vi "Periodic Tasks.vi"(8 "error in":errorcluster) -> ()   [LabVIEW 2023]
doc: "This VI runs in parallel to other tasks. It can contain as many user-defined periodic loops as you need. These can carry out PID or other sorts of timed response."
uses:
  <vilib>/Rock Robotics/WPI/ThirdParty/Phoenix-LabVIEW/Motor Controller/Controls/CTRE_Phoenix_MotorControl_ControlMode.ctl
  <vilib>/Rock Robotics/WPI/Utilities/WPI_GetSetVariantRefNum.vi
  <vilib>/Rock Robotics/Network Tables/NT Read Number.vi
  <vilib>/Rock Robotics/Network Tables/NT Write Boolean.vi
  Robot Global Data.vi
panel:
  out "In Range Speaker Right?":bool=TRUE
  out "In Range Speaker Left?":bool=TRUE
  out "In Range Center?":bool=TRUE
  out "Values":T1
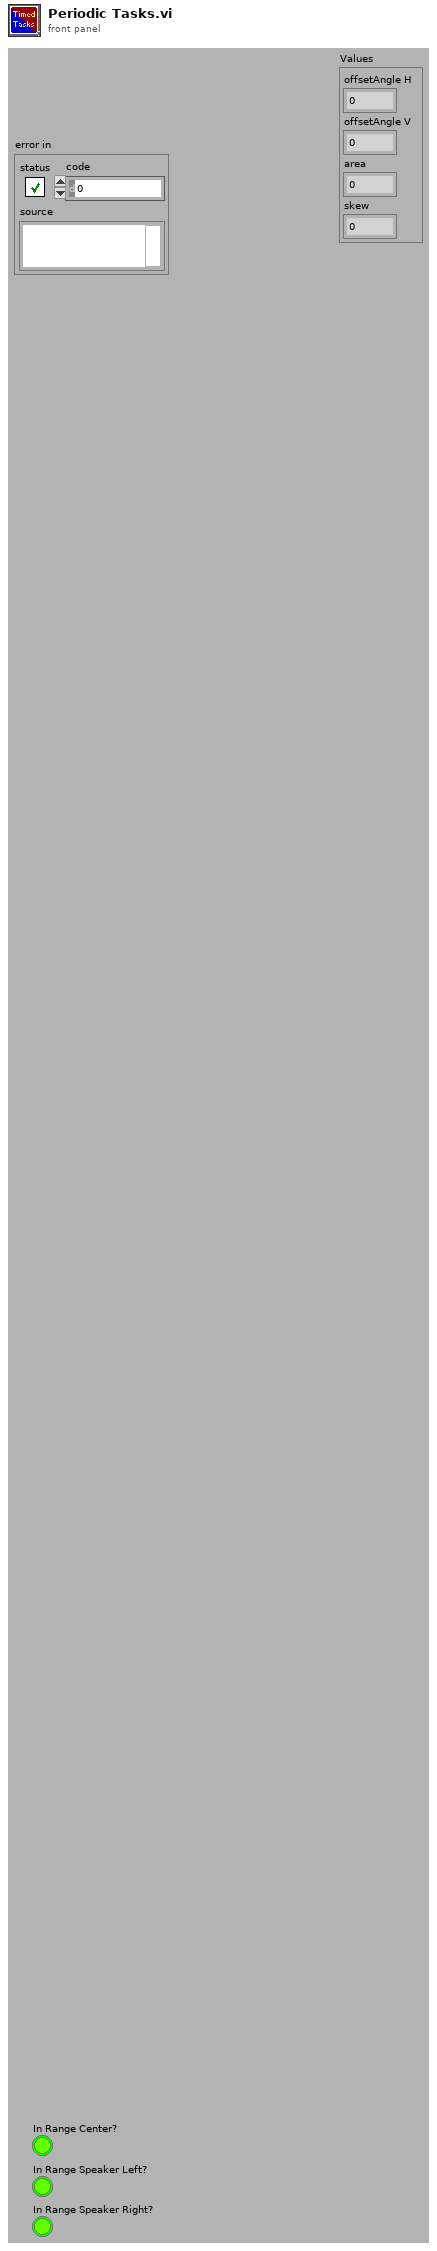
[diagram p1: front panel]
types:
  T1 = cluster{"offsetAngle H":dbl, "offsetAngle V":dbl, "area":dbl, "skew":dbl}
  T2 = typedef "WPI_JoystickDevRef.ctl" = cluster{"Device":T3}
  T3 = typedef "WPI_JoystickDeviceEnum.ctl" = enum16{"USB 0", "USB 1", "USB 2", "USB 3", "USB 4", "USB 5"}
  T4 = typedef "WPI_RobotDriveDevRef.ctl" = cluster{"DevStatus":errorcluster, "Motors[]":T5[], "Square Inputs":bool, "Max Output":dbl}
  T5 = typedef "WPI_MotorControlDeviceRef.ctl" = cluster{"DeviceStatus":errorcluster, "Type":T6, "PWM":cluster{"PWM Channel":T7, "DeadBand":T8}, "CAN":cluster{"Device Number":u8, "SetOutput VI Ref":variant, "GetOutput VI Ref":variant, "Enable VI Ref":variant, "Disable VI Ref":variant, "Data":variant}, "Invert":bool, "DIO PWM":cluster{"PWM \"Enable\" Channel":T7, "DIOChannel":T9, "PWM Rate":dbl}}
  T6 = typedef "WPI_MotorControlType.ctl" = enum16{"PWM", "CAN", "DIO PWM"}
  T7 = typedef "FPGA_DIOPWMChannel.ctl" = enum8{"PWM 0", "PWM 1", "PWM 2", "PWM 3", "PWM 4", "PWM 5", "PWM 6", "PWM 7", "PWM 8", "PWM 9", "PWM MXP 0", "PWM MXP 1", "PWM MXP 2", "PWM MXP 3", "PWM MXP 4", "PWM MXP 5", "PWM MXP 6", "PWM MXP 7", "PWM MXP 8", "PWM MXP 9", "Invalid"}
  T8 = typedef "WPI_PWMDeadband.ctl" = cluster{"Name":string, "maxPositivePwm":i32, "minPositivePwm":i32, "centerPwm":i32, "maxNegativePwm":i32, "minNegativePwm":i32, "angularRange":u16}
  T9 = typedef "FPGA_DIOChannel.ctl" = enum8{"DIO 0", "DIO 1", "DIO 2", "DIO 3", "DIO 4", "DIO 5", "DIO 6", "DIO 7", "DIO 8", "DIO 9", "DIO MXP 0", "DIO MXP 1", "DIO MXP 2", "DIO MXP 3", "DIO MXP 4", "DIO MXP 5", "DIO MXP 6", "DIO MXP 7", "DIO MXP 8", "DIO MXP 9", "DIO MXP 10", "DIO MXP 11", "DIO MXP 12", "DIO MXP 13", "DIO MXP 14", "DIO MXP 15", "SPI Port CS1", "SPI Port CS2", "SPI Port CS3", "SPI Port MISO", "SPI Port MOSI", "Invalid"}
  T10 = cluster{"JoystickDevRef":T2, "RobotDriveDevRef":T4}
  T11 = typedef "CTRE_Phoenix_MotorControl_ControlMode.ctl" = u16
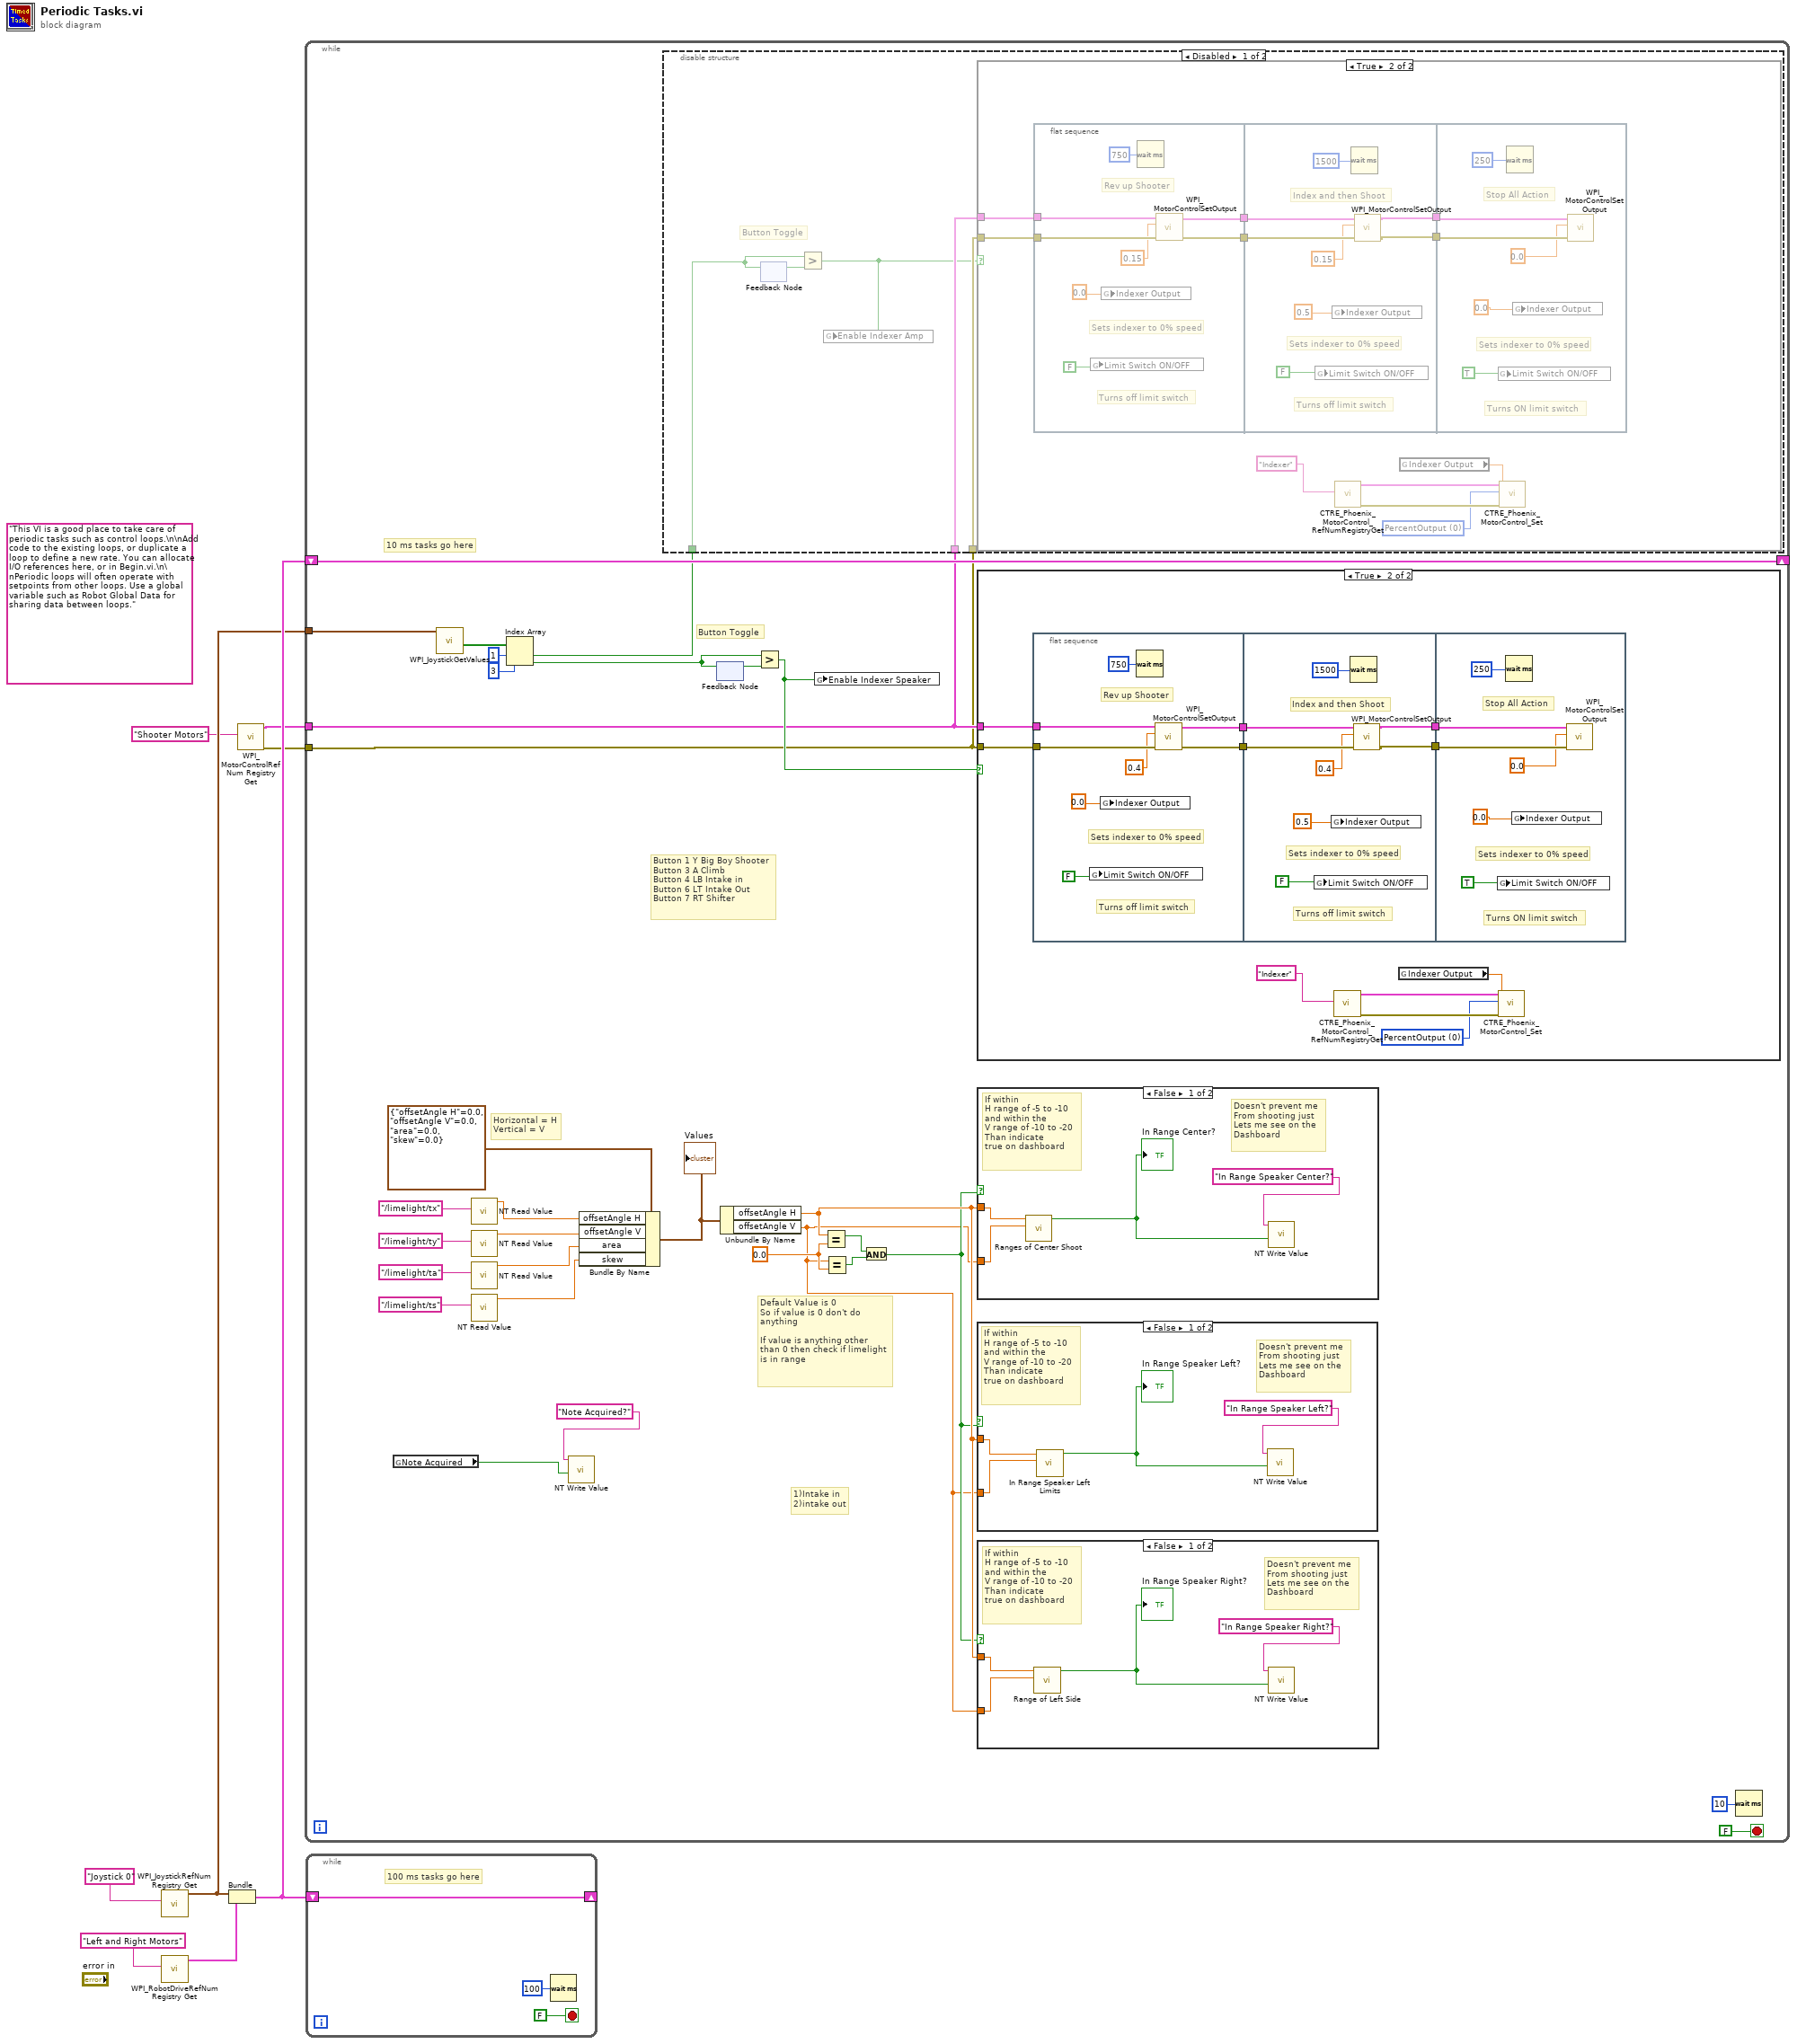
[diagram p0: block diagram]
diagram:
  (unwired) "This VI is a good place to take care of periodic tasks such as control loops.\n\nAdd code to the existing loops, or duplicate a loop to define a new rate. You can allocate I/O references here, or in Begin.vi.\n\nPeriodic loops will often operate with setpoints from other loops. Use a global variable such as Robot Global Data for sharing data between loops."
  n1 = call <vilib>:"WPI_JoystickRefNum Registry Get.vi"("refnum name"="Joystick 0") -> ("JoystickDevRef"=w4:T2)  [unwired: 1 in, 9 out]
  n2 = call <vilib>:"WPI_RobotDriveRefNum Registry Get.vi"("refnum name"="Left and Right Motors") -> ("RobotDriveDevRef"=w6:T4)  [unwired: 1 in, 9 out]
  n3 = Bundle("JoystickDevRef"=w4, "RobotDriveDevRef"=w6) -> (w5:T10)  [unwired: 1 out]
  n4 = call <vilib>:"WPI_MotorControlRefNum Registry Get.vi"("refnum name"="Shooter Motors") -> ("error out"=w1:errorcluster, "MotorControlDevRef"=w2:T5)  [unwired: 9 in]
  n5 = while {
    shift-right: [w37] -> _
    shift-left: w5 -> [w37]
    tunnel: w4 -> [w33]
    tunnel: w2 -> [w15]
    tunnel: w1 -> [w14]
    stop <- FALSE stop-if-true
    w19 = 0.0 ("y")
    # "1)Intake in\n2)intake out"
    # "Default Value is 0\nSo if value is 0 don't do\nanything\n\nIf value is anything other \nthan 0 then check if limelight\nis in range"
    # "Horizontal = H\nVertical = V"
    # "Button 1 Y Big Boy Shooter\nButton 3 A Climb\nButton 4 LB Intake in\nButton 6 LT Intake Out\nButton 7 RT Shifter"
    # "Button Toggle"
    # "10 ms tasks go here"
    n6 = global read "Robot Global Data.vi" "Note Acquired"() -> (w9:bool)
    n7 = call <vilib>:"WPI_JoystickGetValues.vi"("JoystickDevRef"=w33) -> ("Buttons"=w36:bool[])  [unwired: 6 in, 4 out]
    n8 = call-poly <vilib>:"NT Read Value.vi"("name"="/limelight/tx") -> ("value"=w25:dbl)  [unwired: 8 in, 2 out]
    n9 = call-poly <vilib>:"NT Read Value.vi"("name"="/limelight/ty") -> ("value"=w24:dbl)  [unwired: 8 in, 2 out]
    n10 = call-poly <vilib>:"NT Read Value.vi"("name"="/limelight/ta") -> ("value"=w27:dbl)  [unwired: 8 in, 2 out]
    n11 = call-poly <vilib>:"NT Read Value.vi"("name"="/limelight/ts") -> ("value"=w26:dbl)  [unwired: 8 in, 2 out]
    n12 = Index Array(array=w36, index #1=1 ("index"), index #2=3 ("index")) -> (element #1=w12:bool, element #2=w13:bool)
    n13 = call-poly <vilib>:"NT Write Value.vi"("value"=w9, "name"="Note Acquired?") -> ()  [unwired: 9 in, 1 out]
    n14 = Bundle By Name(cluster=T1 {"offsetAngle H"=0.0, "offsetAngle V"=0.0, "area"=0.0, "skew"=0.0}, "offsetAngle H"=w25, "offsetAngle V"=w24, "area"=w27, "skew"=w26) -> (w23:T1)
    "Values" <- w23
    n15 = disable-structure shown="Disabled" {
      disable-tunnel: w15 -> [w44 _]
      disable-tunnel: w14 -> [w43 _]
      disable-tunnel: w12 -> [w41 _]
      frame Disabled {
        # "Button Toggle"
        n16 = feedback #1() -> (w42:bool)  [unwired: 1 in]
        n17 = feedback-in #1(w41) -> ()
        n18 = Greater?(x=w41, y=w42) -> (0:w40:bool)
        n19 = global write "Robot Global Data.vi" "Enable Indexer Amp"(w40) -> ()
        n20 = case shown="True" w40 {
          tunnel: w44 -> [_ w55]
          tunnel: w43 -> [_ w54]
          frame False {
          }
          frame True {
            w46 = T11 0 items=["PercentOutput"=0, "Position"=1, "Velocity"=2, "Current"=3, "Follower"=5, "MotionProfile"=6, "MotionMagic"=7, "MotionProfileArc"=10, "Disabled"=15] ("Control Mode")
            n21 = flat-sequence {
              tunnel: [w60] -> w53
              tunnel: [w59] -> w52
              tunnel: w55 -> [w63]
              tunnel: w54 -> [w62]
              tunnel: w53 -> [w70]
              tunnel: w52 -> [w69]
              tunnel: [w68] -> w51
              tunnel: [w67] -> w50
              tunnel: w51 -> [w77]
              tunnel: w50 -> [w76]
              frame #0 {
                # "Sets indexer to 0% speed"
                # "Rev up Shooter"
                # "Turns off limit switch"
                n22 = global write "Robot Global Data.vi" "Limit Switch ON/OFF"(FALSE ("Limit Switch ON/OFF")) -> ()
                n23 = global write "Robot Global Data.vi" "Indexer Output"(0.0 ("Indexer Output")) -> ()
                n24 = Wait (ms)(milliseconds to wait=u32 750) -> ()  [unwired: 1 out]
                n25 = call <vilib>:"WPI_MotorControlSetOutput.vi"("error in (no error)"=w62, "Output"=0.15, "MotorControlDevRef"=w63) -> ("error out"=w59:errorcluster, "MotorControlDevRef"=w60:T5)  [unwired: 6 in, 1 out]
              }
              frame #1 {
                # "Sets indexer to 0% speed"
                # "Turns off limit switch"
                # "Index and then Shoot"
                n26 = global write "Robot Global Data.vi" "Limit Switch ON/OFF"(FALSE ("Limit Switch ON/OFF")) -> ()
                n27 = global write "Robot Global Data.vi" "Indexer Output"(0.5 ("Indexer Output")) -> ()
                n28 = Wait (ms)(milliseconds to wait=u32 1500) -> ()  [unwired: 1 out]
                n29 = call <vilib>:"WPI_MotorControlSetOutput.vi"("error in (no error)"=w69, "Output"=0.15, "MotorControlDevRef"=w70) -> ("error out"=w67:errorcluster, "MotorControlDevRef"=w68:T5)  [unwired: 6 in, 1 out]
              }
              frame #2 {
                # "Sets indexer to 0% speed"
                # "Turns ON limit switch"
                # "Stop All Action"
                n30 = global write "Robot Global Data.vi" "Limit Switch ON/OFF"(TRUE ("Limit Switch ON/OFF")) -> ()
                n31 = Wait (ms)(milliseconds to wait=u32 250) -> ()  [unwired: 1 out]
                n32 = global write "Robot Global Data.vi" "Indexer Output"(0.0 ("Indexer Output")) -> ()
                n33 = call <vilib>:"WPI_MotorControlSetOutput.vi"("error in (no error)"=w76, "Output"=0.0, "MotorControlDevRef"=w77) -> ()  [unwired: 6 in, 3 out]
              }
            }
            n34 = call <vilib>:"CTRE_Phoenix_MotorControl_RefNumRegistryGet.vi"("refnum name"="Indexer") -> ("error out"=w47:errorcluster, "PhoenixMotorControlDevRef"=w48:T5)  [unwired: 9 in]
            n35 = global read "Robot Global Data.vi" "Indexer Output"() -> (w45:dbl)
            n36 = call <vilib>:"CTRE_Phoenix_MotorControl_Set.vi"("error in (no error)"=w47, "Output"=w45, "Control Mode"=w46, "PhoenixMotorControlDevRef"=w48) -> ()  [unwired: 6 in, 2 out]
          }
        }
      }
      frame Enabled {
      }
    }
    n37 = feedback #2() -> (w34:bool)  [unwired: 1 in]
    n38 = feedback-in #2(w13) -> ()
    n39 = Unbundle By Name(w23) -> ("offsetAngle H"=w22:dbl, "offsetAngle V"=w17:dbl)
    n40 = Greater?(x=w13, y=w34) -> (0:w16:bool)
    n41 = global write "Robot Global Data.vi" "Enable Indexer Speaker"(w16) -> ()
    n42 = Equal?(x=w22, y=w19) -> (x = y?=w21:bool)
    n43 = Equal?(x=w17, y=w19) -> (x = y?=w18:bool)
    n44 = And(x=w21, y=w18) -> (x .and. y?=w20:bool)
    n45 = case shown="True" w16 {
      tunnel: w15 -> [_ w100]
      tunnel: w14 -> [_ w99]
      frame False {
      }
      frame True {
        w91 = T11 0 items=["PercentOutput"=0, "Position"=1, "Velocity"=2, "Current"=3, "Follower"=5, "MotionProfile"=6, "MotionMagic"=7, "MotionProfileArc"=10, "Disabled"=15] ("Control Mode")
        n46 = flat-sequence {
          tunnel: [w105] -> w98
          tunnel: [w104] -> w97
          tunnel: w100 -> [w108]
          tunnel: w99 -> [w107]
          tunnel: w98 -> [w115]
          tunnel: w97 -> [w114]
          tunnel: [w113] -> w96
          tunnel: [w112] -> w95
          tunnel: w96 -> [w122]
          tunnel: w95 -> [w121]
          frame #0 {
            # "Sets indexer to 0% speed"
            # "Rev up Shooter"
            # "Turns off limit switch"
            n47 = global write "Robot Global Data.vi" "Limit Switch ON/OFF"(FALSE ("Limit Switch ON/OFF")) -> ()
            n48 = global write "Robot Global Data.vi" "Indexer Output"(0.0 ("Indexer Output")) -> ()
            n49 = Wait (ms)(milliseconds to wait=u32 750) -> ()  [unwired: 1 out]
            n50 = call <vilib>:"WPI_MotorControlSetOutput.vi"("error in (no error)"=w107, "Output"=0.4, "MotorControlDevRef"=w108) -> ("error out"=w104:errorcluster, "MotorControlDevRef"=w105:T5)  [unwired: 6 in, 1 out]
          }
          frame #1 {
            # "Sets indexer to 0% speed"
            # "Turns off limit switch"
            # "Index and then Shoot"
            n51 = global write "Robot Global Data.vi" "Limit Switch ON/OFF"(FALSE ("Limit Switch ON/OFF")) -> ()
            n52 = global write "Robot Global Data.vi" "Indexer Output"(0.5 ("Indexer Output")) -> ()
            n53 = Wait (ms)(milliseconds to wait=u32 1500) -> ()  [unwired: 1 out]
            n54 = call <vilib>:"WPI_MotorControlSetOutput.vi"("error in (no error)"=w114, "Output"=0.4, "MotorControlDevRef"=w115) -> ("error out"=w112:errorcluster, "MotorControlDevRef"=w113:T5)  [unwired: 6 in, 1 out]
          }
          frame #2 {
            # "Sets indexer to 0% speed"
            # "Turns ON limit switch"
            # "Stop All Action"
            n55 = global write "Robot Global Data.vi" "Limit Switch ON/OFF"(TRUE ("Limit Switch ON/OFF")) -> ()
            n56 = Wait (ms)(milliseconds to wait=u32 250) -> ()  [unwired: 1 out]
            n57 = global write "Robot Global Data.vi" "Indexer Output"(0.0 ("Indexer Output")) -> ()
            n58 = call <vilib>:"WPI_MotorControlSetOutput.vi"("error in (no error)"=w121, "Output"=0.0, "MotorControlDevRef"=w122) -> ()  [unwired: 6 in, 3 out]
          }
        }
        n59 = call <vilib>:"CTRE_Phoenix_MotorControl_RefNumRegistryGet.vi"("refnum name"="Indexer") -> ("error out"=w92:errorcluster, "PhoenixMotorControlDevRef"=w93:T5)  [unwired: 9 in]
        n60 = global read "Robot Global Data.vi" "Indexer Output"() -> (w90:dbl)
        n61 = call <vilib>:"CTRE_Phoenix_MotorControl_Set.vi"("error in (no error)"=w92, "Output"=w90, "Control Mode"=w91, "PhoenixMotorControlDevRef"=w93) -> ()  [unwired: 6 in, 2 out]
      }
    }
    n62 = case shown="False" w20 {
      tunnel: w22 -> [w84 _]
      tunnel: w17 -> [w83 _]
      frame False {
        # "Doesn't prevent me \nFrom shooting just\nLets me see on the\nDashboard"
        # "If within \nH range of -5 to -10\nand within the \nV range of -10 to -20 \nThan indicate \ntrue on dashboard"
        n63 = call "In Range Speaker Left Limits.vi"("offsetAngle V"=w83, "offsetAngle H"=w84) -> ("Boolean"=w82:bool)  [unwired: 9 in]
        "In Range Speaker Left?" <- w82
        n64 = call-poly <vilib>:"NT Write Value.vi"("value"=w82, "name"="In Range Speaker Left?") -> ()  [unwired: 9 in, 1 out]
      }
      frame True {
      }
    }
    n65 = case shown="False" w20 {
      tunnel: w22 -> [w88 _]
      tunnel: w17 -> [w87 _]
      frame False {
        # "Doesn't prevent me \nFrom shooting just\nLets me see on the\nDashboard"
        # "If within \nH range of -5 to -10\nand within the \nV range of -10 to -20 \nThan indicate \ntrue on dashboard"
        n66 = call "Ranges of Center Shoot.vi"("offsetAngle V"=w87, "offsetAngle H"=w88) -> ("Boolean"=w86:bool)  [unwired: 9 in]
        "In Range Center?" <- w86
        n67 = call-poly <vilib>:"NT Write Value.vi"("value"=w86, "name"="In Range Speaker Center?") -> ()  [unwired: 9 in, 1 out]
      }
      frame True {
      }
    }
    n68 = case shown="False" w20 {
      tunnel: w22 -> [w80 _]
      tunnel: w17 -> [w79 _]
      frame False {
        # "Doesn't prevent me \nFrom shooting just\nLets me see on the\nDashboard"
        # "If within \nH range of -5 to -10\nand within the \nV range of -10 to -20 \nThan indicate \ntrue on dashboard"
        n69 = call "Range of Left Side.vi"("offsetAngle V"=w79, "offsetAngle H"=w80) -> ("Boolean"=w78:bool)  [unwired: 9 in]
        "In Range Speaker Right?" <- w78
        n70 = call-poly <vilib>:"NT Write Value.vi"("value"=w78, "name"="In Range Speaker Right?") -> ()  [unwired: 9 in, 1 out]
      }
      frame True {
      }
    }
    n71 = Wait (ms)(milliseconds to wait=u32 10) -> ()  [unwired: 1 out]
  }
  n72 = while {
    shift-right: [w123] -> _
    shift-left: w5 -> [w123]
    stop <- FALSE stop-if-true
    # "100 ms tasks go here"
    n73 = Wait (ms)(milliseconds to wait=u32 100) -> ()  [unwired: 1 out]
  }
